vi "Get Memory Statistics.vi"(3 "error in (no error)":errorcluster, 5 "get storage info? (T)":bool=TRUE) -> (0 "error out":errorcluster, 1 "App Memory Statistics":T2, 2 "VI Memory Statistics":T3(array[cluster]))   [LabVIEW 2021, in "Utilities.lvlib"]
doc: "Gathers information about all VIs currently in memory.\n\nFor each VI, it produces this information:\n1) The path to the VI's file.\n2) The size of the data space attached to the VI's front panel. A re-entrant VI has a data space for each usage of the VI. Therefore, this number is not a true reflection of the amount of data a VI is responsible for.\n3&4) The size of the VI's front panel and the number of objects in it; both are zero if the front panel is not currently in memory.\n5&6) Same as above for the block diagram\n7) size of the code generated for this VI.\n8) the VI's description.\n9) The VI's handle.\n10) the indices into the raw data array of this VI's callers\n11) the indices into the raw data array of this VI's callees (subVIs)."
uses:
  Utilities.lvlib
panel:
  in  "?":T1
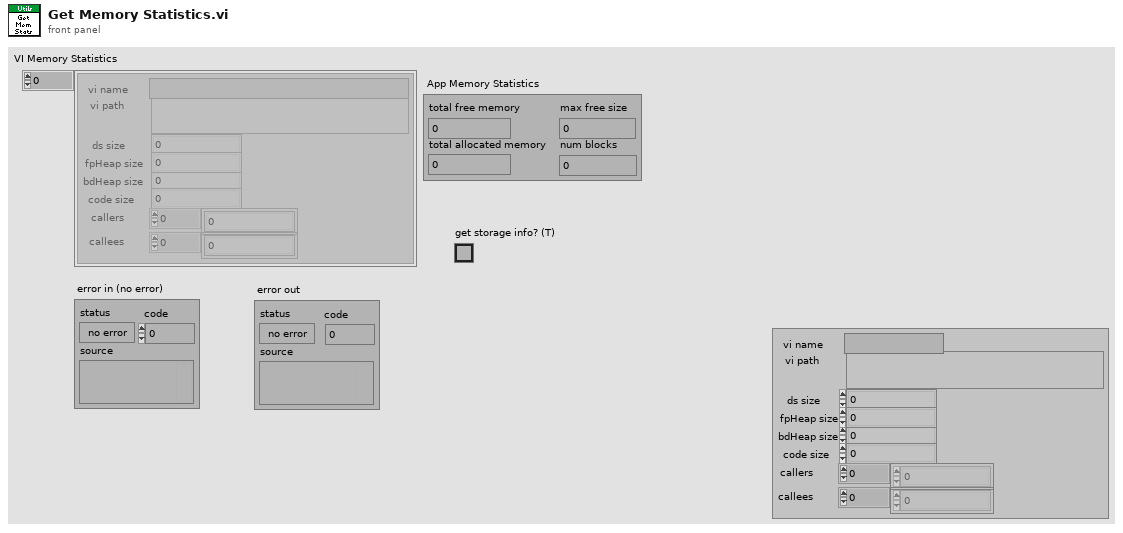
[diagram p1: front panel]
types:
  T1 = cluster{"vi name":string, "vi path":path, "ds size":i32, "fpHeap size":i32, "bdHeap size":i32, "code size":i32, "callers":u32[], "callees":u32[]}
  T2 = cluster{"total free memory":i32, "max free size":i32, "total allocated memory":i32, "num blocks":i32}
  T3 = cluster{"vi name":string, "vi path":path, "ds size":i32, "fpHeap size":i32, "bdHeap size":i32, "code size":i32, "callers":u32[], "callees":u32[]}[]
  T4 = cluster{"totalFreeSize":i64, "maxFreeSize":i64, "nFreeblocks":i64, "totAllocSize":i64, "maxAllocSize":i64, "nPointers":i64, "nUnlockedHdls":i64, "nLockedHdls":i64, "reserved1":i32, "reserved2":i32, "reserved3":i32, "reserved4":i32}
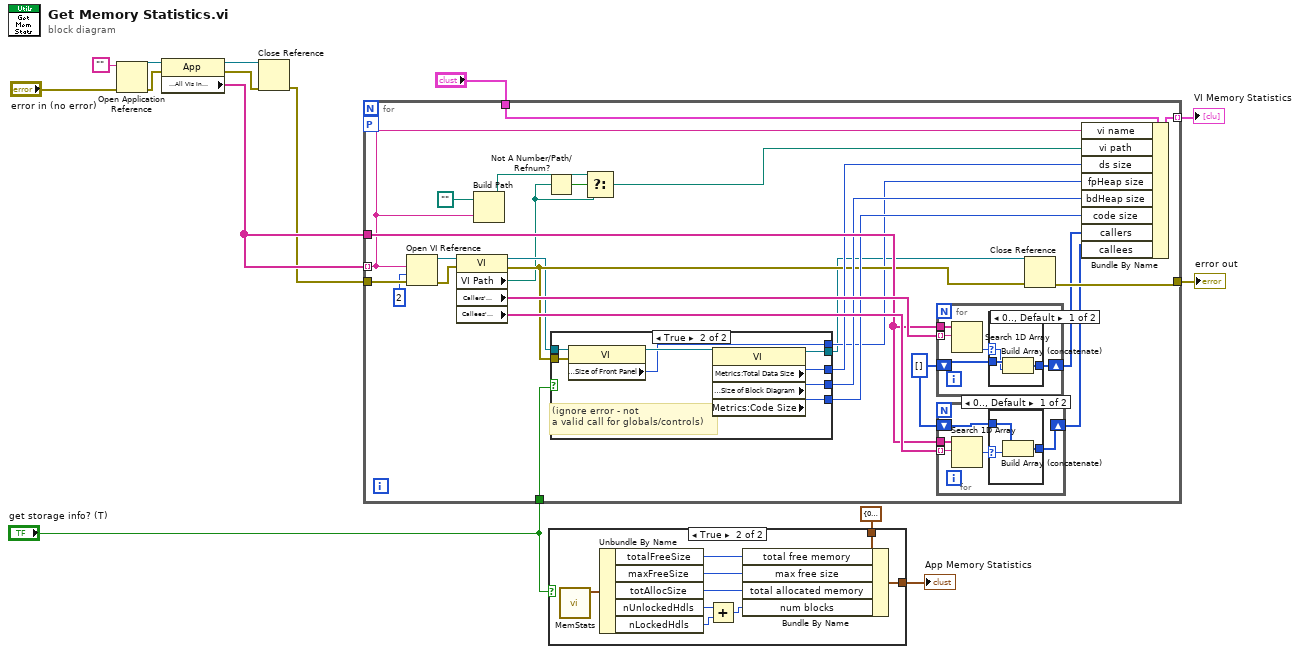
[diagram p0: block diagram]
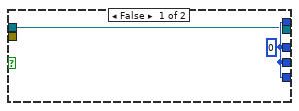
[diagram p2: hidden frame]
diagram:
  n1 = Open Application Reference(8:"error in (no error)", 11:"" ("machine name (\"\":  open local reference)")) -> (0:w13:errorcluster, 3:w14:refnum<vi>)  [unwired: 2 in]
  n2 = property class="App"(reference=w14, error in=w13) -> (reference out=w12:refnum<vi>, error out=w11:errorcluster, "Application:All VIs In Memory"=w9:string[])
  n3 = Close Reference(reference=w12, error in (no error)=w11) -> (error out=w7:errorcluster)
  n4 = for {
    tunnel: w9 -> [w18] mode=indexing
    tunnel: "?" -> [w39]
    tunnel: [w38] -> w8 mode=indexing
    tunnel: w9 -> [w35]
    tunnel: "get storage info? (T)" -> [w27]
    tunnel: w7 -> [w34]
    tunnel: [w33] -> w5
    workers-P: _ -> [_]
    w23 = i32[] []
    n5 = Open VI Reference(vi path=w18, options=2, error in (no error)=w34) -> (vi reference=w41:refnum<vi>, error out=w40:errorcluster)  [unwired: 3 in]
    n6 = property class="VI"(reference=w41, error in=w40) -> (reference out=w26:refnum<vi>, error out=w29:errorcluster, "VI Path"=w20:path, "Callers' Names"=w37:string[], "Callees' Names"=w36:string[])
    n7 = Build Path(base path=path "", name or relative path=w18) -> (appended path=w17:path)
    n8 = Not A Number/Path/Refnum?(number/path/refnum=w20) -> (NaN/Path/Refnum?=w21:bool)
    n9 = case shown="True" w27 {
      tunnel: [w43 w51] -> w32
      tunnel: [w43 w50] -> w31
      tunnel: [w43 w49] -> w30
      tunnel: w26 -> [w42 w47]
      tunnel: w29 -> [_ w46]
      tunnel: [w43 w45] -> w28
      tunnel: [w42 w44] -> w25
      frame False {
        w43 = u32 0 ("Metric.CodeSize")
      }
      frame True {
        # "(ignore error - not\na valid call for globals/controls)"
        n10 = property class="VI"(reference=w47, error in=w46) -> (reference out=w48:refnum<vi>, "Metrics:Size of Front Panel"=w45:u32)  [unwired: 1 out]
        n11 = property class="VI"(reference=w48) -> (reference out=w44:refnum<vi>, "Metrics:Total Data Size"=w50:u32, "Metrics:Size of Block Diagram"=w49:u32, "Metrics:Code Size"=w51:u32)  [unwired: 1 in, 1 out]
      }
    }
    n12 = Select(t=w17, s=w21, f=w20) -> (s? t:f=w19:path)
    n13 = for {
      tunnel: w37 -> [w65] mode=indexing
      tunnel: w35 -> [w64]
      shift-right: [w61] -> w24
      shift-left: w23 -> [w62]
      n14 = Search 1D Array(1D array=w64, element=w65) -> (index of element=w63:i32)  [unwired: 1 in]
      n15 = case shown="0.., Default" w63 {
        selector: w63 -> [w67 _]
        tunnel: w62 -> [w68 w69]
        tunnel: [w66 w69] -> w61
        frame 0.., Default {
          n16 = Build Array (concatenate)(w68, w67) -> (w66:i32[])
        }
        frame -1 {
        }
      }
    }
    n17 = for {
      tunnel: w36 -> [w56] mode=indexing
      tunnel: w35 -> [w55]
      shift-right: [w53] -> w22
      shift-left: w23 -> [w52]
      n18 = Search 1D Array(1D array=w55, element=w56) -> (index of element=w54:i32)  [unwired: 1 in]
      n19 = case shown="0.., Default" w54 {
        selector: w54 -> [w59 _]
        tunnel: [w58 w60] -> w53
        tunnel: w52 -> [w57 w60]
        frame 0.., Default {
          n20 = Build Array (concatenate)(w57, w59) -> (w58:i32[])
        }
        frame -1 {
        }
      }
    }
    n21 = Close Reference(reference=w25, error in (no error)=w29) -> (error out=w33:errorcluster)
    n22 = Bundle By Name(cluster=w39, "vi name"=w18, "vi path"=w19, "ds size"=w31, "fpHeap size"=w28, "bdHeap size"=w30, "code size"=w32, "callers"=w24, "callees"=w22) -> (w38:T1)
  }
  "VI Memory Statistics" <- w8
  "error out" <- w5
  n23 = case shown="True" "get storage info? (T)" {
    tunnel: [w70 w72] -> w3
    tunnel: T2 {"total free memory"=0, "max free size"=0, "total allocated memory"=0, "num blocks"=0} ("App Memory Statistics") -> [w70 w71]
    frame False {
    }
    frame True {
      n24 = call <vilib>:"MemStats.vi"() -> ("AZ memStats"=w79:T4)  [unwired: 5 in, 2 out]
      n25 = Unbundle By Name(w79) -> ("totalFreeSize"=w78:i64, "maxFreeSize"=w77:i64, "totAllocSize"=w76:i64, "nUnlockedHdls"=w75:i64, "nLockedHdls"=w74:i64)
      n26 = Add(x=w75, y=w74) -> (x+y=w73:i64)
      n27 = Bundle By Name(cluster=w71, "total free memory"=w78, "max free size"=w77, "total allocated memory"=w76, "num blocks"=w73) -> (w72:T2)
    }
  }
  "App Memory Statistics" <- w3
